vi "Write Elements.vi"(8 "error in (no error)":errorcluster, 10 "Elements":refnum<class "Geometric.lvclass">[](array[class]), 11 "Structure.lvclass in":refnum<class "Structure.lvclass">) -> (0 "error out":errorcluster, 3 "Structure.lvclass out":refnum<class "Structure.lvclass">)   [LabVIEW 2019, in "Structure.lvclass"]
uses:
  Structure.lvclass
  Structure.lvclass/Structure.ctl
  Elements/Geometric.lvclass
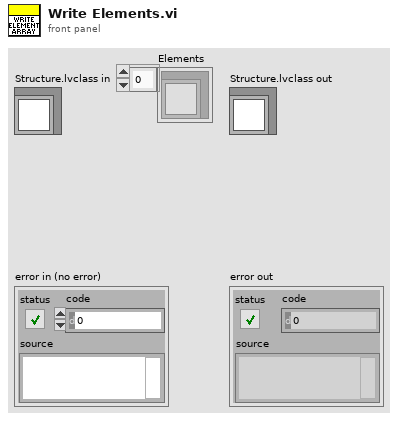
[diagram p1: front panel]
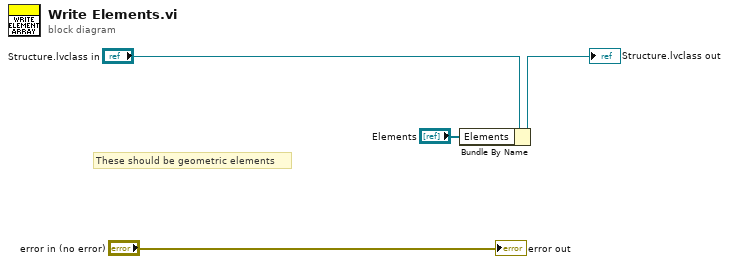
[diagram p0: block diagram]
diagram:
  # "These should be geometric elements"
  n1 = Bundle By Name(cluster="Structure.lvclass in", "Elements"="Elements") -> (→"Structure.lvclass out":refnum<class "Structure.lvclass">)
  "error out" <- "error in (no error)"
